vi "Publish.vi"(8 "error in (no error)":errorcluster, 9 "body":u8[](array[numeric]), 10 "header":T1, 11 "publisher in":refnum<class "IcmMessagePublisher.lvclass">) -> (0 "error out":errorcluster, 3 "publisher out":refnum<class "IcmMessagePublisher.lvclass">)   [LabVIEW 2017, in "IcmMessagePublisher.lvclass"]
doc: "Publishes a message to the message bus."
uses:
  <vilib>/addons/InsightCM/MessageBus/MessagePublisher/IcmMessagePublisher.lvclass
  <vilib>/addons/InsightCM/MessageBus/Base/controls/MessageHeader.ctl
  <vilib>/addons/InsightCM/MessageBus/Base/controls/KeyValuePair.ctl
  <vilib>/addons/InsightCM/MessageBus/MessagePublisher/IcmMessagePublisher.lvclass/IcmMessagePublisher.ctl
  C:/Program Files (x86)/National Instruments/LabVIEW 2017/vi.lib/addons/InsightCM/Binaries/LabviewMessageAdapter.dll
  Binaries/LabviewMessageAdapter.dll
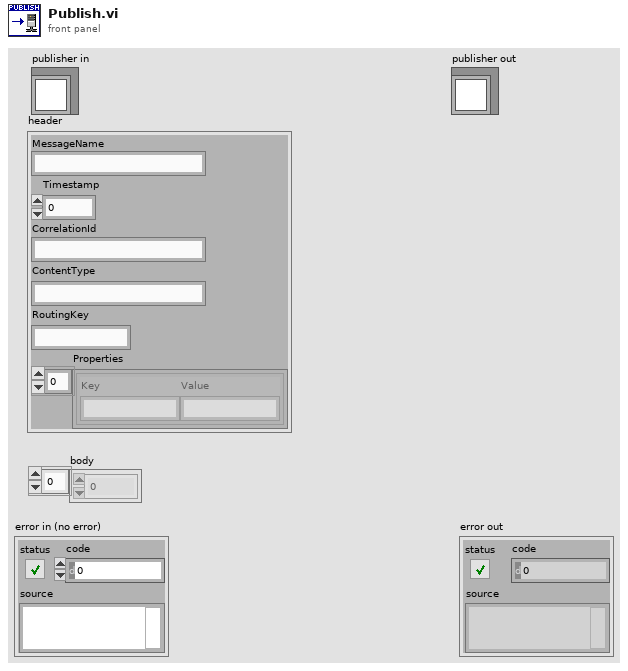
[diagram p1: front panel]
types:
  T1 = typedef "MessageHeader.ctl" = cluster{"MessageName":string, "Timestamp":i64, "CorrelationId":string, "ContentType":string, "RoutingKey":string, "Properties":T2[]}
  T2 = typedef "KeyValuePair.ctl" = cluster{"Key":string, "Value":string}
  T3 = typedef "MessagePublisherDvr.ctl" = refnum<data-value>
  T4 = typedef "MessagePublisherData.ctl" = cluster{"Publisher":refnum<k24>}
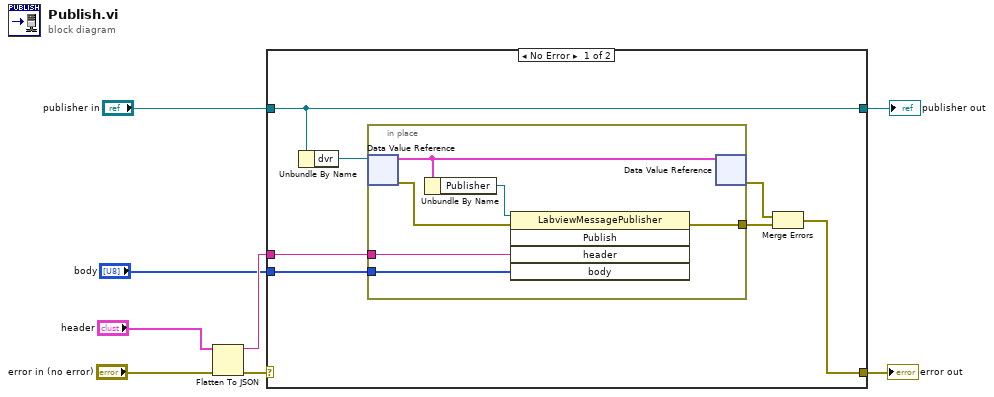
[diagram p0: block diagram]
diagram:
  n1 = Flatten To JSON(anything="header", error in (no error)="error in (no error)") -> (JSON string=w4:string, 11:w6:errorcluster)  [unwired: 1 in]
  n2 = case shown="No Error" w6 {
    selector: w6 -> [_ w23]
    tunnel: [w11 w23] -> w8
    tunnel: [w15 w22] -> w1
    tunnel: "publisher in" -> [w15 w22]
    tunnel: w4 -> [w10 _]
    tunnel: "body" -> [w9 _]
    frame No Error {
      n3 = Unbundle By Name(w15) -> ("dvr"=w14:T3)
      n4 = in-place {
        in-place-border: [w18] -> w12
        in-place-border: w10 -> [w17]
        in-place-border: w9 -> [w16]
        n5 = in-place-dvr #1(w14) -> (w21:T4, w19:errorcluster)
        n6 = Unbundle By Name(w21) -> ("Publisher"=w20:refnum<k24>)
        n7 = invoke class="LabviewMessagePublisher" method="Publish"(reference=w20, error in=w19, "header"=w17, "body"=w16) -> (error out=w18:errorcluster)  [unwired: 1 in, 4 out]
        n8 = in-place-dvr #1(w21) -> (w13:errorcluster)  [unwired: 1 out]
      }
      n9 = Merge Errors(w13, w12) -> (w11:errorcluster)
    }
    frame Error {
    }
  }
  "error out" <- w8
  "publisher out" <- w1
